vi "MeasDetails.vi"(8 "error in":errorcluster, 10 "Active measurement":string, 11 "gRPC session in":T1) -> (0 "error out":errorcluster, 3 "gRPC session out":T1)   [LabVIEW 2021, in "dcvmDPI_AD7606B_clientImpl.lvlib"]
uses:
  dcvmDPI_AD7606B_clientImpl.lvlib
  <vilib>/gRPC/LabVIEW gRPC Library/Shared/grpcId.ctl
  dcvmDPI_AD7606B_client/RPC Messages/dcvmDPI_MeasurementRequest.ctl
  dcvmDPI_AD7606B_client/dcvmDPI_AD7606B_client.lvlib
  <vilib>/gRPC/LabVIEW gRPC Library/grpc-lvsupport-release.lvlib
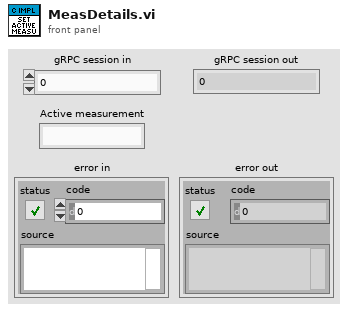
[diagram p1: front panel]
types:
  T1 = typedef "grpc-lvsupport-release.lvlib/grpcId.ctl" = u64
  T2 = typedef "dcvmDPI_AD7606B_client.lvlib/dcvmDPI_MeasurementRequest.ctl" = cluster{"measurement":string}
  T3 = typedef "dcvmDPI_AD7606B_client.lvlib/dcvmDPI_MeasurementResponse.ctl" = cluster{"error":T4}
  T4 = typedef "dcvmDPI_AD7606B_client.lvlib/dcvmDPI_ErrorResponse.ctl" = cluster{"error_number":i32, "error_description":string}
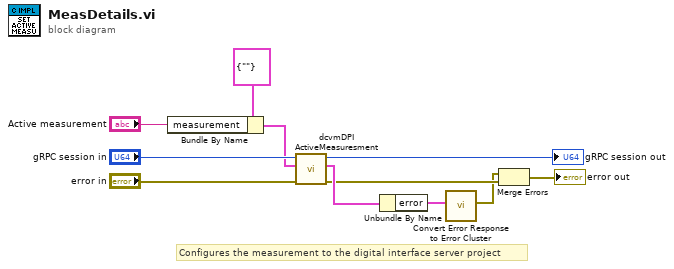
[diagram p0: block diagram]
diagram:
  # "Configures the measurement to the digital interface server project"
  n1 = Bundle By Name(cluster=T2 {"measurement"=""} ("Request Data"), "measurement"="Active measurement") -> (w8:T2)
  n2 = call "dcvmDPI ActiveMeasuresment.vi"("error in"="error in", "Request Data"=w8, "gRPC ID"="gRPC session in") -> ("error out"=w3:errorcluster, "Response Data"=w5:T3, "gRPC ID out"=→"gRPC session out":T1)  [unwired: 6 in]
  n3 = Unbundle By Name(w5) -> ("error"=w4:T4)
  n4 = call "Convert Error Response to Error Cluster.vi"("Error response"=w4) -> ("error out"=w2:errorcluster)  [unwired: 10 in]
  n5 = Merge Errors(w2, w3) -> (→"error out":errorcluster)
